vi "题目1.vi"   [LabVIEW 2017]
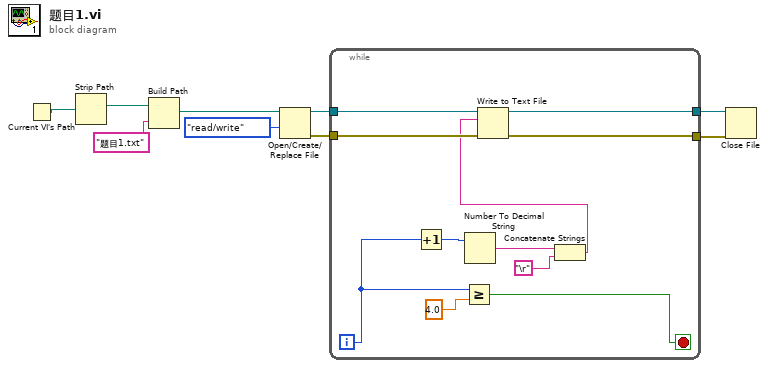
[diagram p0: block diagram]
diagram:
  n1 = Current VI's Path() -> (path=w9:path)
  n2 = Strip Path(path=w9) -> (stripped path=w8:path)  [unwired: 1 out]
  n3 = Build Path(base path=w8, name or relative path="题目1.txt" ("名称或相对路径")) -> (appended path=w6:path)
  n4 = Open/Create/Replace File(file path (use dialog)=w6, access (0:read/write)=enum16{"read/write", "read-only", "write-only"}."read/write" ("权限(0:read/write)")) -> (refnum out=w5:refnum<file>, error out=w4:errorcluster)  [unwired: 4 in, 1 out]
  n5 = while {
    tunnel: w5 -> [w13]
    tunnel: w4 -> [w14]
    tunnel: [w12] -> w3
    tunnel: [w11] -> w2
    i -> [w16]
    stop <- w15 stop-if-true
    n6 = Increment(x=w16) -> (x+1=w18:i32)
    n7 = Greater Or Equal?(x=w16, y=4.0) -> (x >= y?=w15:bool)
    n8 = Number To Decimal String(number=w18) -> (decimal integer string=w17:string)  [unwired: 1 in]
    n9 = Concatenate Strings(w17, "\r" ("字符串")) -> (w10:string)
    n10 = Write to Text File(file (use dialog)=w13, text=w10, error in=w14) -> (refnum out=w12:refnum<file>, error out=w11:errorcluster)  [unwired: 1 in, 1 out]
  }
  n11 = Close File(refnum=w3, error in=w2) -> ()  [unwired: 2 out]
